vi "Get_nice_dimensions_for_displayed_cage.vi"(3 "Cage Dims.":T3={"Width, mm"=180.0, "Height, mm"=180.0}, 4 "Draw Area Size":T2={"Width, pix"=480, "Height, pix"=480}, 5 "Target scale factor the max displayed cage size":dbl=0.96 min=0.01 max=10.0 step=0.01) -> (2 "Image Geometry and Scilng info":T1)   [LabVIEW 2018, in "Cage Diagram.lvlib"]
uses:
  Cage Diagram.lvlib
  Typedefs/CTL_Cage_External_dimensions.ctl
  SubVi's/Controls/CTL_Draw_Area_Size.ctl
  Typedefs/CTL_Image_Scaling_info.ctl
  Common_Resources.lvlib
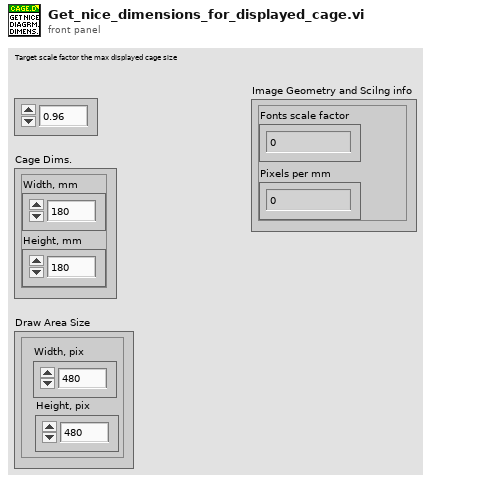
[diagram p1: front panel]
types:
  T1 = typedef "Cage Diagram.lvlib/CTL_Image_Scaling_info.ctl" = cluster{"Fonts scale factor":dbl, "Pixels per mm":dbl}
  T2 = typedef "Common_Resources.lvlib/CTL_Draw_Area_Size.ctl" = cluster{"Width, pix":i32, "Height, pix":i32}
  T3 = typedef "Cage Diagram.lvlib/CTL_Cage_External_dimensions.ctl" = cluster{"Width, mm":dbl, "Height, mm":dbl}
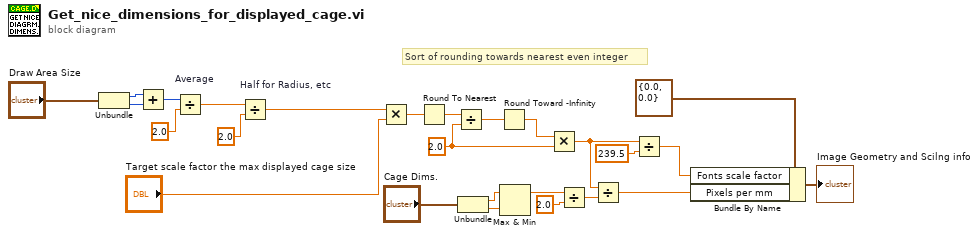
[diagram p0: block diagram]
diagram:
  w9 = 2.0 ("y")
  # "Sort of rounding towards nearest even integer"
  n1 = Unbundle("Draw Area Size") -> ("Width, pix"=w15:i32, "Height, pix"=w14:i32)
  n2 = Add(x=w15, y=w14) -> (x+y=w16:i32)
  n3 = Divide "Average"(x=w16, y=2.0) -> (x/y=w19:dbl)
  n4 = Divide "Half for Radius, etc"(x=w19, y=2.0) -> (x/y=w25:dbl)
  n5 = Multiply(x=w25, y="Target scale factor the max displayed cage size") -> (x*y=w13:dbl)
  n6 = Round To Nearest(number=w13) -> (nearest integer value=w12:dbl)
  n7 = Divide(x=w12, y=w9) -> (x/y=w11:dbl)
  n8 = Unbundle("Cage Dims.") -> ("Width, mm"=w8:dbl, "Height, mm"=w7:dbl)
  n9 = Round Toward -Infinity(1:w11) -> (0:w10:dbl)
  n10 = Max & Min(x=w8, y=w7) -> (max(x,y)=w6:dbl)  [unwired: 1 out]
  n11 = Multiply(x=w10, y=w9) -> (x*y=w3:dbl)
  n12 = Divide(x=w6, y=2.0) -> (x/y=w22:dbl)
  n13 = Divide(x=w3, y=w22) -> (x/y=w2:dbl)
  n14 = Divide(x=w3, y=239.5) -> (x/y=w4:dbl)
  n15 = Bundle By Name(cluster=T1 {"Fonts scale factor"=0.0, "Pixels per mm"=0.0} ("Image Geometry and Scaling parameters"), "Fonts scale factor"=w4, "Pixels per mm"=w2) -> (→"Image Geometry and Scilng info":T1)
